vi "FPGAcode2_old.vi"() -> ()   [LabVIEW 2015]
uses:
  <vilib>/Platform/TimedLoop/XDataNode/timing_clust.ctl
  <vilib>/Platform/TimedLoop/XDataNode/nitl_modes.ctl
  <vilib>/Platform/TimedLoop/XDataNode/wakeup.ctl
  Filter Cutoffs.ctl
  Filter Logic In.ctl
  <vilib>/rvi/Emulation/niFpgaGetClockAttributes.vi
  <vilib>/rvi/Emulation/niFpgaSctlEmulationGetInTimedLoop.vi
  <vilib>/rvi/Emulation/niFpgaEmulationReportErrorSimple.vi
  <vilib>/rvi/Emulation/niFpgaProcessEmulError.vi
  <vilib>/rvi/eio/common/nirviEmuTemplateMethod_errors.vi
  <vilib>/rvi/Emulation/niFpgaCriticalErrorInLSC.vi
  <vilib>/eio/EIONode/EIONode.xnode
  <vilib>/Platform/TimedLoop/XDataNode/XDataNode.xnode
  <vilib>/Platform/TimedLoop/XDataNode/XDNodeRunTimeDep.lvlib
panel:
  out "Detector 3 Correlation 7":i16
  out "Detector 3 Correlation 6":i16
  out "Detector 3 Correlation 5":i16
  out "Detector 3 Correlation 4":i16
  out "Detector 3 Correlation 3":i16
  out "Detector 3 Correlation 2":i16
  out "Detector 3 Correlation 1":i16
  out "Detector 1 Correlation 7":i16
  out "Detector 1 Correlation 6":i16
  out "Detector 1 Correlation 5":i16
  out "Detector 1 Correlation 4":i16
  out "Detector 1 Correlation 3":i16
  out "Detector 1 Correlation 2":i16
  out "Detector 1 Correlation 1":i16
  in  "Filter threshold 7":i32=1000
  in  "Filter threshold 6":i32=1000
  in  "Filter threshold 5":i32=1000
  in  "Filter threshold 4":i32=1000
  in  "Filter threshold 3":i32=1000
  in  "Filter threshold 2":i32=1000
  in  "Filter threshold 1":i32=1000
  out "Del Armed":bool
  out "Armed":bool
  out "Delay":bool
  out "Plates":bool
  in  "Reset One Shot":bool
  in  "One Shot":bool
  in  "High Charge Limit":i16
  in  "Low Charge Limit":i16
  in  "High Velocity Count":i32
  in  "Low Velocity Count":i32
  in  "High Mass Limit":i64
  in  "Low Mass Limit":i64
  in  "Mult1":fxp<+,16,7>
  out "IO Module\\AI 0":i16
  out "IO Module\\AI 1":i16
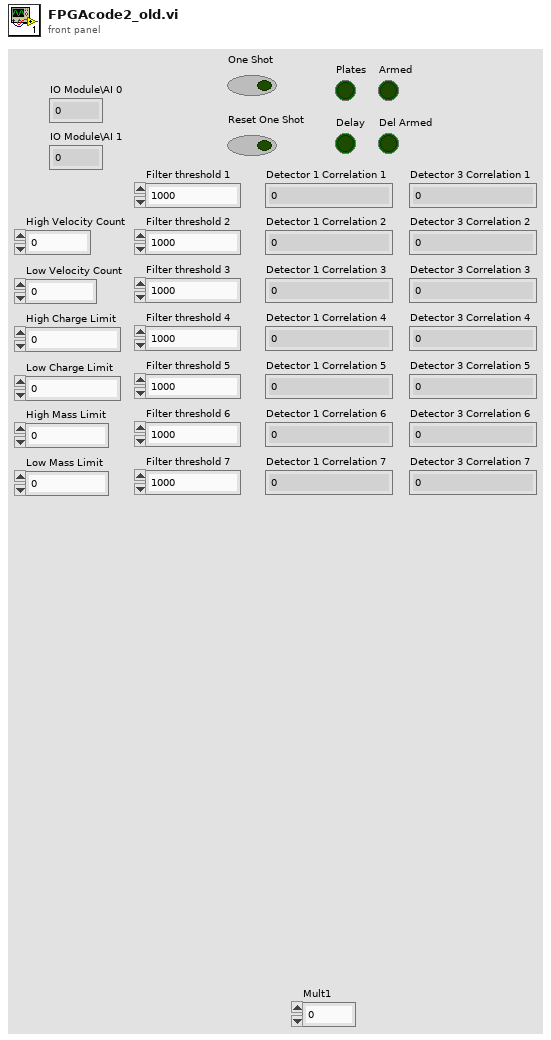
[diagram p1: front panel]
types:
  T1 = typedef "Filter Cutoffs.ctl" = cluster{"High Cutoff":i32, "Low Cutoff":i32}
  T2 = typedef "XDNodeRunTimeDep.lvlib/timing_clust.ctl" = cluster{"Expected End [f-1]":u64, "Actual End [f-1]":u64, "Finished Late? [f-1]":bool, "Expected End [i-1]":u64, "Actual End [i-1]":u64, "Finished Late? [i-1]":bool, "Expected Start [i]":u64, "Actual Start [i]":u64, "Expected Start [f]":u64, "Actual Start [f]":u64, "Source Name":string, "Structure Name":string, "Period":i64, "Deadline":i64, "Offset":i64, "Start":i64, "Priority":i32, "Timeout":i32, "Mode":T3, "Wakeup Reason":T4, "Error":errorcluster, "Source Type":string, "Secondary Source Type":string, "Global End Time":u64, "Global Start Time":u64, "Frame Duration":u64, "Iteration Duration":u64, "Assigned CPU":i32, "I/O Scan Engine Mode":u32}
  T3 = typedef "XDNodeRunTimeDep.lvlib/nitl_modes.ctl" = enum32{"No Change", "Process missed periods, maintain original phase", "Discard missed periods, maintain original phase", "Process missed periods, ignore original phase", "Discard missed periods, ignore original phase"}
  T4 = typedef "XDNodeRunTimeDep.lvlib/wakeup.ctl" = enum32{"Normal", "Aborted", "Asynchronous wakeup", "Timing source error", "Timed loop error", "Timeout"}
  T5 = typedef "Filter Logic In.ctl" = cluster{"Old Average":i16, "New Average":i16, "Current State":u8, "Detector 1 Correlation":i16, "Detector 3 Correlation":i16, "Velocity Count":i32, "Detector Counter in":i32, "Timeout Count in":u32, "Measured Charge in":i32, "Filter Threshold":i32, "High Correlation in":i32, "Offset":i32, "Offset Average":i32, "Measured Velocity In":i32, "Mult1":fxp<+,16,7>, "Delay1 In":i32, "Final Delay Count In":u16}
  T6 = typedef "Limits.ctl" = cluster{"High Charge Limit":i16, "Low Charge Limit":i16, "Time Out Limit":i32, "High Velocity Count":i32, "Low Velocity Count":i32, "Sampling Rate":fxp<+,30,25>, "High Mass Limit":i64, "Low Mass Limit":i64}
  T7 = cluster{"Average Out":i32, "Next State":u8, "Velocity Count out":i32, "Detector counter out":i32, "Timeout count out":u32, "Measured Charge Out":i32, "High Correlation Out":i32, "Plates":bool, "Offset Out":i32, "Measured Velocity Out":i32, "Final Delay Count Out":u16, "Out1":bool, "Delay1":i32}
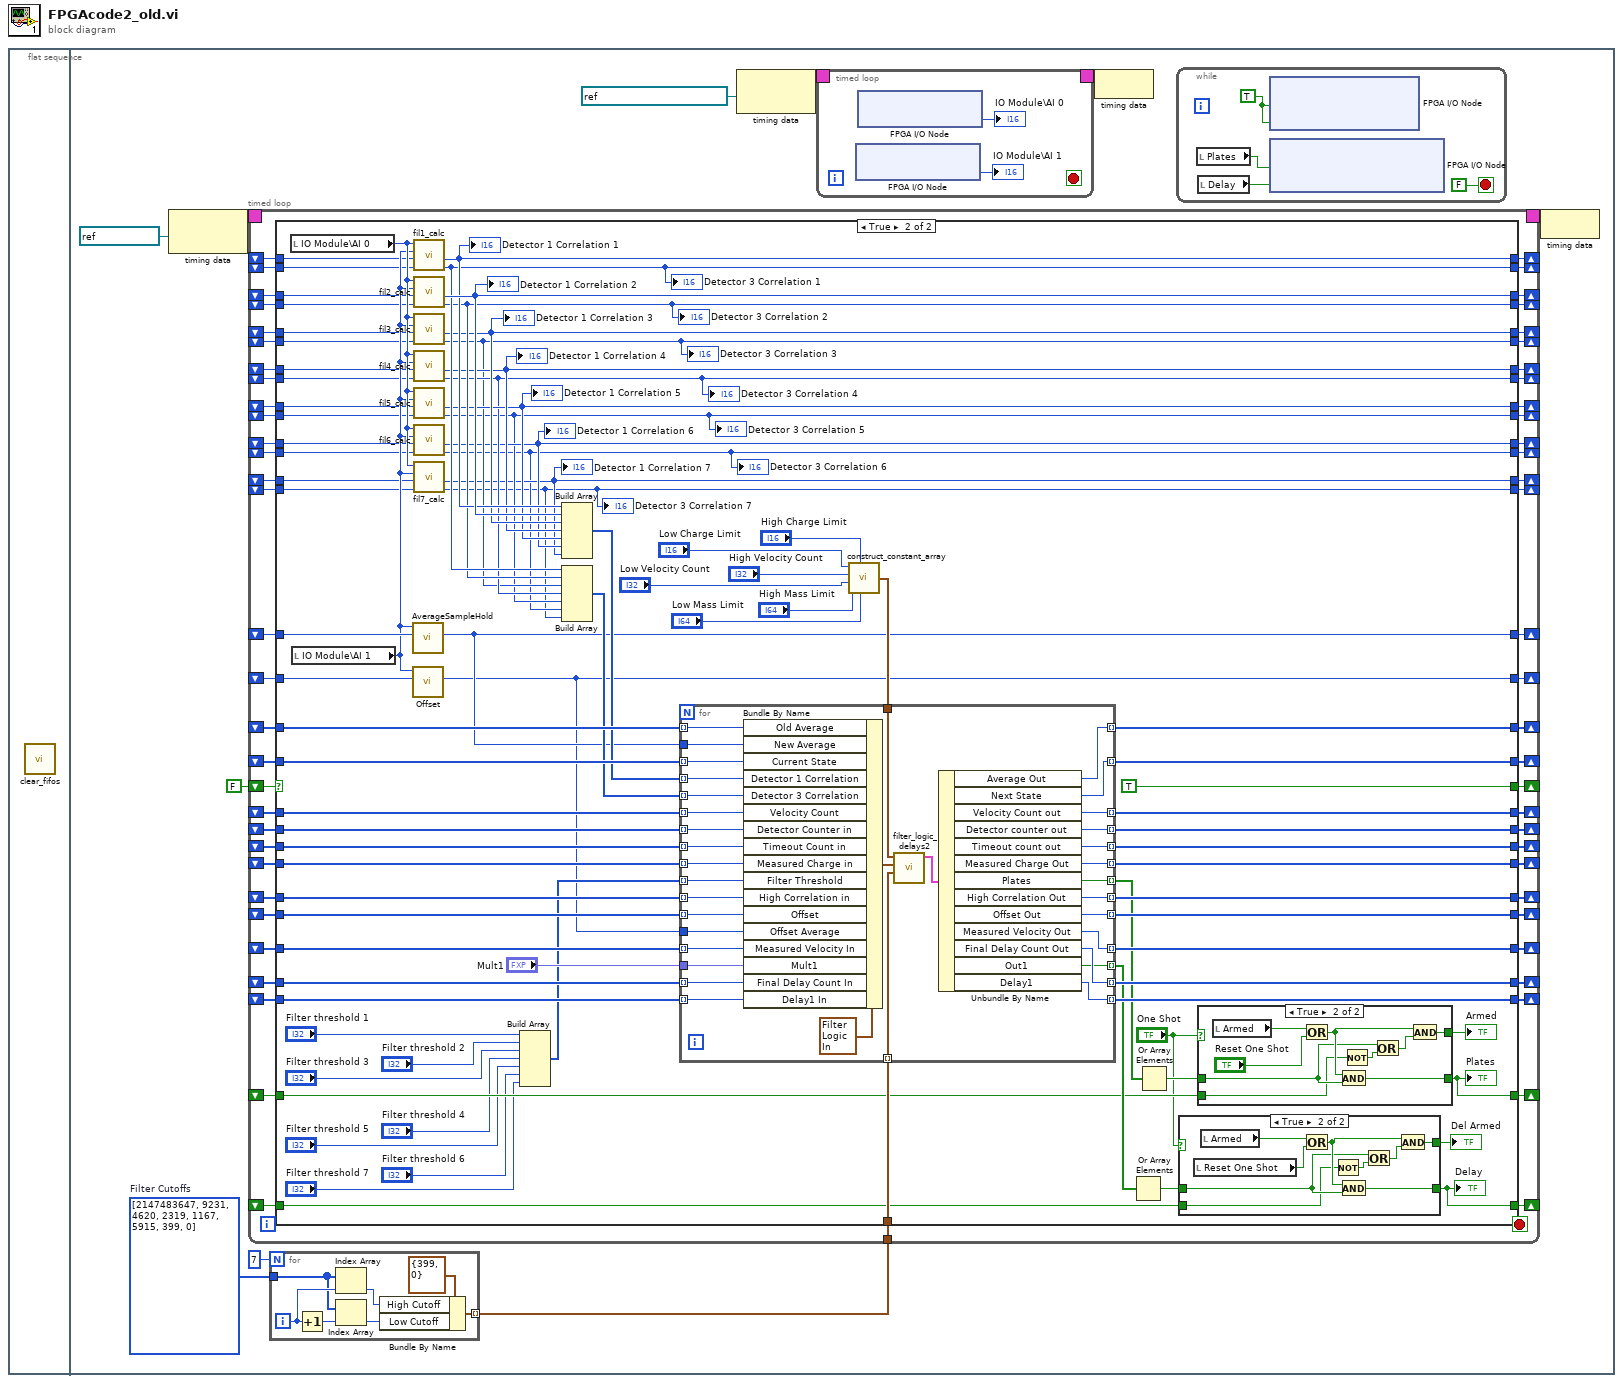
[diagram p0: block diagram]
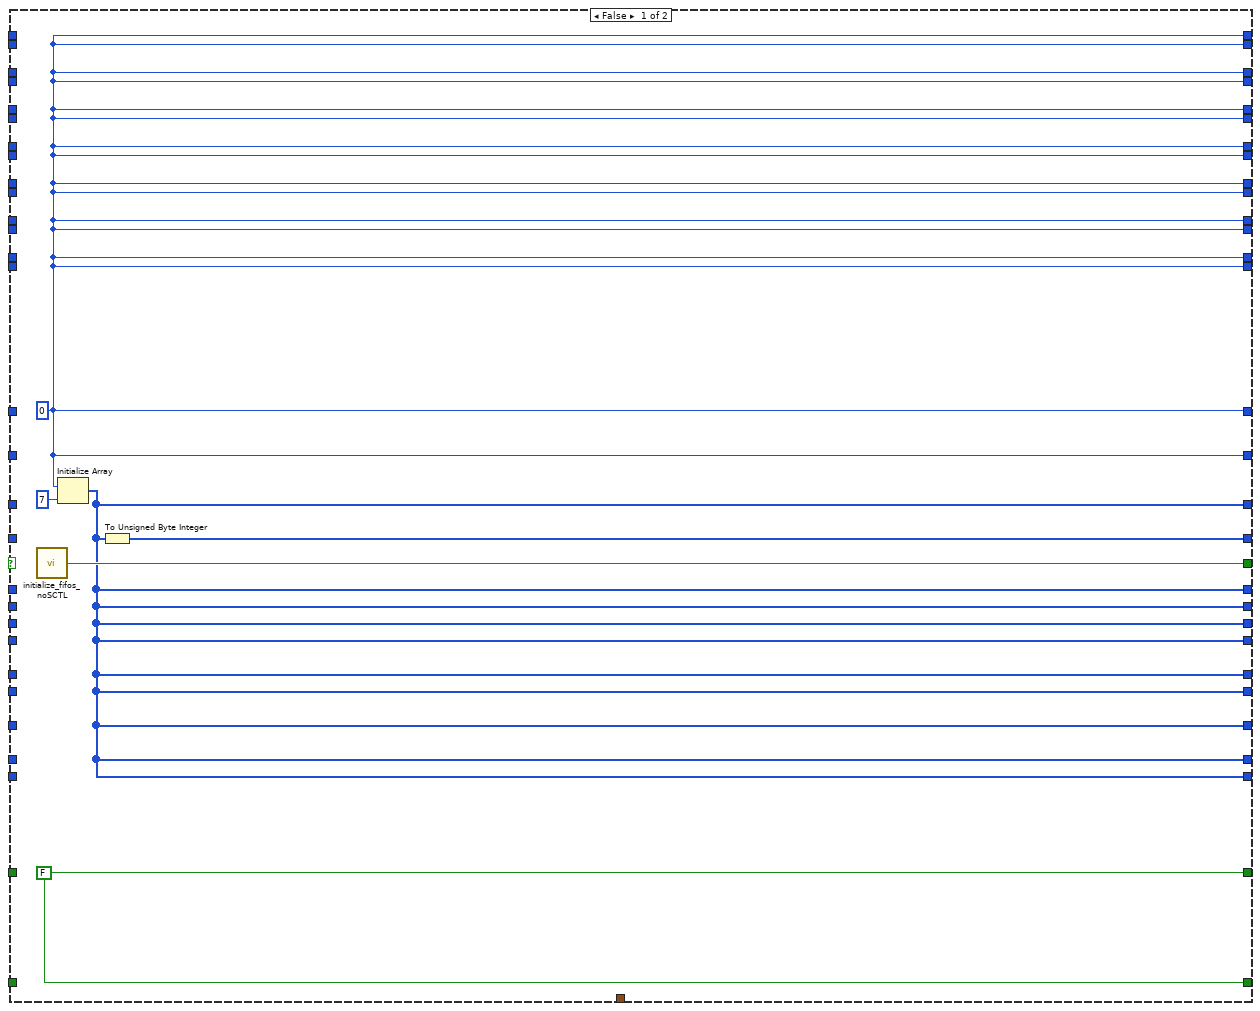
[diagram p2: hidden frame]
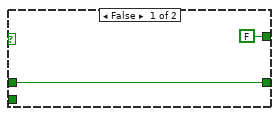
[diagram p3: hidden frame]
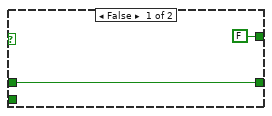
[diagram p4: hidden frame]
diagram:
  n1 = flat-sequence {
    frame #0 {
      n2 = call "clear_fifos.vi"() -> ()  [unwired: 1 in]
    }
    frame #1 {
      w1 = i32[] [2147483647, 9231, 4620, 2319, 1167, 5915, 399, 0]  # Filter Cutoffs
      n3 = node-c288(refnum<k21> "26.67MHz" ("Source Name")) -> (w10:T2)
      n4 = for {
        N: 7 -> [_]
        tunnel: [w16] -> w3 mode=indexing
        tunnel: w1 -> [w13]
        i -> [w15]
        n5 = Increment(x=w15) -> (x+1=w14:i32)
        n6 = Index Array(array=w13, index=w15) -> (element=w11:i32)
        n7 = Index Array(array=w13, index=w14) -> (element=w12:i32)
        n8 = Bundle By Name(cluster=T1 {"High Cutoff"=399, "Low Cutoff"=0} ("Filter Specific Constants"), "High Cutoff"=w11, "Low Cutoff"=w12) -> (w16:T1)
      }
      n9 = timed-loop {
        timing: w10 -> [_]
        timing-out: [_] -> w9
        shift-right: [w89] -> _
        shift-left: FALSE -> [w90]
        tunnel: w3 -> [w88]
        shift-right: [w86] -> _
        shift-left: _ -> [w87]
        shift-right: [w84] -> _
        shift-left: _ -> [w85]
        shift-right: [w82] -> _
        shift-left: _ -> [w83]
        shift-right: [w68] -> _
        shift-left: _ -> [w81]
        shift-right: [w79] -> _
        shift-left: _ -> [w80]
        shift-right: [w77] -> _
        shift-left: _ -> [w78]
        shift-right: [w67] -> _
        shift-left: _ -> [w76]
        shift-right: [w66] -> _
        shift-left: _ -> [w75]
        shift-right: [w62] -> _
        shift-left: _ -> [w74]
        shift-right: [w72] -> _
        shift-left: _ -> [w73]
        shift-right: [w65] -> _
        shift-left: _ -> [w71]
        shift-right: [w64] -> _
        shift-left: _ -> [w70]
        shift-right: [w63] -> _
        shift-left: _ -> [w69]
        shift-right: [w61] -> _
        shift-left: _ -> [w60]
        shift-right: [w58] -> _
        shift-left: _ -> [w59]
        shift-right: [w57] -> _
        shift-left: _ -> [w56]
        shift-right: [w55] -> _
        shift-left: _ -> [w54]
        shift-right: [w53] -> _
        shift-left: _ -> [w49]
        shift-right: [w52] -> _
        shift-left: _ -> [w48]
        shift-right: [w51] -> _
        shift-left: _ -> [w47]
        shift-right: [w50] -> _
        shift-left: _ -> [w46]
        shift-right: [w45] -> _
        shift-left: _ -> [w37]
        shift-right: [w44] -> _
        shift-left: _ -> [w36]
        shift-right: [w43] -> _
        shift-left: _ -> [w35]
        shift-right: [w42] -> _
        shift-left: _ -> [w30]
        shift-right: [w41] -> _
        shift-left: _ -> [w34]
        shift-right: [w40] -> _
        shift-left: _ -> [w31]
        shift-right: [w39] -> _
        shift-left: _ -> [w33]
        shift-right: [w38] -> _
        shift-left: _ -> [w32]
        stop <- _ stop-if-true
        n10 = case shown="True" w90 {
          tunnel: [w96 TRUE] -> w89
          tunnel: w88 -> [_ w182]
          tunnel: w87 -> [_ w181]
          tunnel: [w93 w180] -> w86
          tunnel: w85 -> [_ w179]
          tunnel: [w91 w112] -> w84
          tunnel: w83 -> [_ w177]
          tunnel: [w94 w176] -> w82
          tunnel: w81 -> [_ w175]
          tunnel: w80 -> [_ w174]
          tunnel: [w93 w173] -> w79
          tunnel: w78 -> [_ w172]
          tunnel: [w93 w171] -> w77
          tunnel: w76 -> [_ w170]
          tunnel: w75 -> [_ w169]
          tunnel: w74 -> [_ w168]
          tunnel: w73 -> [_ w167]
          tunnel: [w91 w111] -> w72
          tunnel: w71 -> [_ w166]
          tunnel: w70 -> [_ w165]
          tunnel: w69 -> [_ w164]
          tunnel: [w93 w163] -> w68
          tunnel: [w93 w162] -> w67
          tunnel: [w93 w161] -> w66
          tunnel: [w93 w160] -> w65
          tunnel: [w93 w159] -> w64
          tunnel: [w93 w158] -> w63
          tunnel: [w93 w157] -> w62
          tunnel: [w95 w151] -> w61
          tunnel: w60 -> [_ w152]
          tunnel: w59 -> [_ w148]
          tunnel: [w95 w147] -> w58
          tunnel: [w91 w97] -> w57
          tunnel: w56 -> [_ w126]
          tunnel: [w91 w99] -> w55
          tunnel: w54 -> [_ w125]
          tunnel: [w91 w98] -> w53
          tunnel: [w91 w101] -> w52
          tunnel: [w91 w100] -> w51
          tunnel: [w91 w104] -> w50
          tunnel: w49 -> [_ w124]
          tunnel: w48 -> [_ w123]
          tunnel: w47 -> [_ w122]
          tunnel: w46 -> [_ w121]
          tunnel: [w91 w103] -> w45
          tunnel: [w91 w105] -> w44
          tunnel: [w91 w102] -> w43
          tunnel: [w91 w106] -> w42
          tunnel: [w91 w107] -> w41
          tunnel: [w91 w110] -> w40
          tunnel: [w91 w108] -> w39
          tunnel: [w91 w109] -> w38
          tunnel: w37 -> [_ w120]
          tunnel: w36 -> [_ w119]
          tunnel: w35 -> [_ w118]
          tunnel: w34 -> [_ w117]
          tunnel: w33 -> [_ w116]
          tunnel: w32 -> [_ w115]
          tunnel: w31 -> [_ w114]
          tunnel: w30 -> [_ w113]
          frame False {
            w95 = FALSE
            w91 = i16 0 ("Output New Average")
            n11 = call "initialize_fifos_noSCTL.vi"() -> ("Output State"=w96:bool)
            n12 = Initialize Array(w91, 7 ("dimension size")) -> (w93:i16[])
            n13 = To Unsigned Byte Integer(number=w93) -> (unsigned 8bit integer=w94:u8[])
          }
          frame True {
            n14 = local read "IO Module\\AI 0"() -> (w138:i16)
            n15 = local read "IO Module\\AI 1"() -> (w137:i16)
            n16 = call "AverageSampleHold.vi"("Previous Average"=w179, "Input Value"=w137) -> ("Output New Average"=w112:i16)  [unwired: 9 in]
            n17 = call "Offset.vi"("Previous Average"=w167, "Input Value"=w137) -> ("Output New Average"=w111:i16)  [unwired: 9 in]
            n18 = call "fil1_calc.vi"("Detector 3 Correlation In"=w116, "Detector 1 Correlation In"=w115, "AI1"=w137, "AI0"=w138) -> ("Detector 3 Correlation Out"=w108:i16, "Detector 1 Correlation Out"=w109:i16)  [unwired: 4 in]
            "Detector 1 Correlation 1" <- w109
            "Detector 3 Correlation 1" <- w108
            n19 = call "fil2_calc.vi"("Detector 3 Correlation In"=w117, "Detector 1 Correlation In"=w114, "AI1"=w137, "AI0"=w138) -> ("Detector 3 Correlation Out"=w107:i16, "Detector 1 Correlation Out"=w110:i16)  [unwired: 4 in]
            "Detector 1 Correlation 2" <- w110
            "Detector 3 Correlation 2" <- w107
            n20 = call "fil3_calc.vi"("Detector 3 Correlation In"=w118, "Detector 1 Correlation In"=w113, "AI1"=w137, "AI0"=w138) -> ("Detector 3 Correlation Out"=w102:i16, "Detector 1 Correlation Out"=w106:i16)  [unwired: 4 in]
            "Detector 1 Correlation 3" <- w106
            "Detector 3 Correlation 3" <- w102
            n21 = call "fil4_calc.vi"("Detector 3 Correlation In"=w120, "Detector 1 Correlation In"=w119, "AI1"=w137, "AI0"=w138) -> ("Detector 3 Correlation Out"=w103:i16, "Detector 1 Correlation Out"=w105:i16)  [unwired: 4 in]
            "Detector 1 Correlation 4" <- w105
            "Detector 3 Correlation 4" <- w103
            n22 = call "fil5_calc.vi"("Detector 3 Correlation In"=w122, "Detector 1 Correlation In"=w121, "AI1"=w137, "AI0"=w138) -> ("Detector 3 Correlation Out"=w100:i16, "Detector 1 Correlation Out"=w104:i16)  [unwired: 4 in]
            "Detector 1 Correlation 5" <- w104
            "Detector 3 Correlation 5" <- w100
            n23 = call "fil6_calc.vi"("Detector 3 Correlation In"=w124, "Detector 1 Correlation In"=w123, "AI1"=w137, "AI0"=w138) -> ("Detector 3 Correlation Out"=w98:i16, "Detector 1 Correlation Out"=w101:i16)  [unwired: 4 in]
            "Detector 1 Correlation 6" <- w101
            "Detector 3 Correlation 6" <- w98
            n24 = call "fil7_calc.vi"("Detector 3 Correlation In"=w126, "Detector 1 Correlation In"=w125, "AI1"=w137, "AI0"=w138) -> ("Detector 3 Correlation Out"=w97:i16, "Detector 1 Correlation Out"=w99:i16)  [unwired: 4 in]
            "Detector 1 Correlation 7" <- w99
            "Detector 3 Correlation 7" <- w97
            n25 = Build Array("Filter threshold 1", "Filter threshold 2", "Filter threshold 3", "Filter threshold 4", "Filter threshold 5", "Filter threshold 6", "Filter threshold 7") -> (w127:i32[])
            n26 = Build Array(w109, w110, w106, w105, w104, w101, w99) -> (w136:i16[])
            n27 = Build Array(w108, w107, w102, w103, w100, w98, w97) -> (w135:i16[])
            n28 = call "construct_constant_array.vi"("Low Mass Limit"="Low Mass Limit", "High Charge Limit"="High Charge Limit", "High Mass Limit"="High Mass Limit", "Low Velocity Count"="Low Velocity Count", "High Velocity Count"="High Velocity Count", "Low Charge Limit"="Low Charge Limit") -> ("Limits"=w178:T6)
            n29 = for {
              tunnel: w136 -> [w209] mode=indexing
              tunnel: w135 -> [w208] mode=indexing
              tunnel: w182 -> [w238] mode=indexing
              tunnel: w181 -> [w235] mode=indexing
              tunnel: [w236] -> w180 mode=indexing
              tunnel: w178 -> [w234]
              tunnel: w177 -> [w233] mode=indexing
              tunnel: [w232] -> w176 mode=indexing
              tunnel: w175 -> [w231] mode=indexing
              tunnel: w174 -> [w230] mode=indexing
              tunnel: [w229] -> w173 mode=indexing
              tunnel: w172 -> [w228] mode=indexing
              tunnel: [w227] -> w171 mode=indexing
              tunnel: w170 -> [w226] mode=indexing
              tunnel: w169 -> [w225] mode=indexing
              tunnel: w168 -> [w224] mode=indexing
              tunnel: w166 -> [w223] mode=indexing
              tunnel: w127 -> [w222] mode=indexing
              tunnel: w165 -> [w221] mode=indexing
              tunnel: w164 -> [w220] mode=indexing
              tunnel: [w219] -> w163 mode=indexing
              tunnel: [w218] -> w162 mode=indexing
              tunnel: [w217] -> w161 mode=indexing
              tunnel: [w216] -> w160 mode=indexing
              tunnel: [w213] -> w159 mode=indexing
              tunnel: [w215] -> w158 mode=indexing
              tunnel: [w214] -> w157 mode=indexing
              tunnel: [w212] -> w156 mode=indexing
              tunnel: [w211] -> w155 mode=indexing
              tunnel: "Mult1" -> [w210]
              tunnel: w112 -> [w207]
              tunnel: w111 -> [w206]
              n30 = Bundle By Name(cluster=T5 {"Old Average"=0, "New Average"=0, "Current State"=0, "Detector 1 Correlation"=0, "Detector 3 Correlation"=0, "Velocity Count"=0, "Detector Counter in"=0, "Timeout Count in"=0, "Measured Charge in"=0, "Filter Threshold"=0, "High Correlation in"=0, "Offset"=0, "Offset Average"=0, "Measured Velocity In"=0, "Mult1"=0.0, "Delay1 In"=0, "Final Delay Count In"=0} ("Variables Cluster"), "Old Average"=w235, "New Average"=w207, "Current State"=w233, "Detector 1 Correlation"=w209, "Detector 3 Correlation"=w208, "Velocity Count"=w231, "Detector Counter in"=w226, "Timeout Count in"=w225, "Measured Charge in"=w223, "Filter Threshold"=w222, "High Correlation in"=w221, "Offset"=w220, "Offset Average"=w206, "Measured Velocity In"=w224, "Mult1"=w210, "Final Delay Count In"=w228, "Delay1 In"=w230) -> (w239:T5)
              n31 = call "filter_logic_delays2.vi"("Filter Limits"=w238, "Variables Cluster"=w239, "Limits Cluster"=w234) -> ("Output Cluster"=w237:T7)  [unwired: 8 in]
              n32 = Unbundle By Name(w237) -> ("Average Out"=w236:i32, "Next State"=w232:u8, "Velocity Count out"=w219:i32, "Detector counter out"=w218:i32, "Timeout count out"=w217:u32, "Measured Charge Out"=w216:i32, "Plates"=w212:bool, "High Correlation Out"=w213:i32, "Offset Out"=w215:i32, "Measured Velocity Out"=w214:i32, "Final Delay Count Out"=w227:u16, "Out1"=w211:bool, "Delay1"=w229:i32)
            }
            n33 = Or Array Elements(Boolean array=w155) -> (logical OR=w150:bool)
            n34 = Or Array Elements(Boolean array=w156) -> (logical OR=w154:bool)
            n35 = case shown="True" "One Shot" {
              tunnel: [w185 w191] -> w147
              tunnel: w150 -> [w185 w188]
              tunnel: [FALSE w193] -> w146
              tunnel: w148 -> [_ w187]
              frame False {
              }
              frame True {
                n36 = local read "Reset One Shot"() -> (w186:bool)
                n37 = local read "Armed"() -> (w194:bool)
                n38 = Or(x=w194, y=w186) -> (x .or. y?=w192:bool)
                n39 = Not(x=w187) -> (.not. x?=w189:bool)
                n40 = And(x=w192, y=w188) -> (x .and. y?=w191:bool)
                n41 = Or(x=w188, y=w189) -> (x .or. y?=w190:bool)
                n42 = And(x=w192, y=w190) -> (x .and. y?=w193:bool)
              }
            }
            "Delay" <- w147
            "Del Armed" <- w146
            n43 = case shown="True" "One Shot" {
              tunnel: [w196 w201] -> w151
              tunnel: w154 -> [w196 w198]
              tunnel: [FALSE w203] -> w153
              tunnel: w152 -> [_ w197]
              frame False {
              }
              frame True {
                n44 = local read "Armed"() -> (w205:bool)
                n45 = Or(x=w205, y="Reset One Shot") -> (x .or. y?=w202:bool)
                n46 = And(x=w202, y=w198) -> (x .and. y?=w201:bool)
                n47 = Not(x=w197) -> (.not. x?=w199:bool)
                n48 = Or(x=w198, y=w199) -> (x .or. y?=w200:bool)
                n49 = And(x=w202, y=w200) -> (x .and. y?=w203:bool)
              }
            }
            "Plates" <- w151
            "Armed" <- w153
          }
        }
      }
      n50 = node-c288(refnum<k21> "IO Module\\Data Clock" ("Source Name")) -> (w7:T2)
      n51 = timed-loop {
        timing: w7 -> [_]
        timing-out: [_] -> w6
        stop <- _ stop-if-true
        n52 = xnode "FPGA I/O Node"() -> ("IO Module\\AI 1"=→"IO Module\\AI 1":i16)  [unwired: 1 in, 1 out]
        n53 = xnode "FPGA I/O Node"() -> ("IO Module\\AI 0"=→"IO Module\\AI 0":i16)  [unwired: 1 in, 1 out]
      }
      n54 = node-c288(w6) -> ()
      n55 = while {
        stop <- FALSE stop-if-true
        w29 = TRUE ("IO Module\\PFI Enable")
        n56 = local read "Plates"() -> (w27:bool)
        n57 = local read "Delay"() -> (w26:bool)
        n58 = xnode "FPGA I/O Node"("IO Module\\PFI 0 WE"=w29, "IO Module\\PFI 1 WE"=w29) -> ()  [unwired: 2 in, 2 out]
        n59 = xnode "FPGA I/O Node"("IO Module\\PFI 0 Wr Data"=w27, "IO Module\\PFI 1 Wr Data"=w26) -> ()  [unwired: 2 in, 2 out]
      }
      n60 = node-c288(w9) -> ()
    }
  }
